vi "Reto2.vi"() -> ()   [LabVIEW 2018]
uses:
  <vilib>/Platform/TimedLoop/XDataNode/timing_clust.ctl
  <vilib>/Platform/TimedLoop/XDataNode/nitl_modes.ctl
  <vilib>/Platform/TimedLoop/XDataNode/wakeup.ctl
  <vilib>/platform/TimedLoop/XDataNode/XDataNode.xnode
  <vilib>/Platform/TimedLoop/XDataNode/XDNodeRunTimeDep.lvlib
panel:
  out "Waveform Chart":dbl(graph)
  in  "x":dbl min=0.0 max=100.0 step=10.0
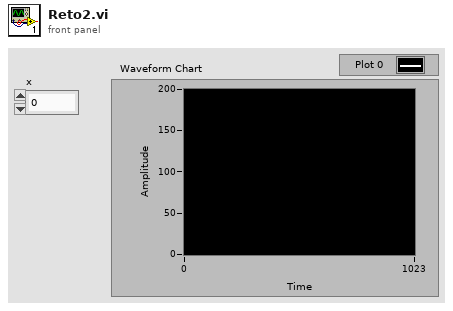
[diagram p1: front panel]
types:
  T1 = typedef "XDNodeRunTimeDep.lvlib/timing_clust.ctl" = cluster{"Expected End [f-1]":u64, "Actual End [f-1]":u64, "Finished Late? [f-1]":bool, "Expected End [i-1]":u64, "Actual End [i-1]":u64, "Finished Late? [i-1]":bool, "Expected Start [i]":u64, "Actual Start [i]":u64, "Expected Start [f]":u64, "Actual Start [f]":u64, "Source Name":string, "Structure Name":string, "Period":i64, "Deadline":i64, "Offset":i64, "Start":i64, "Priority":i32, "Timeout":i32, "Mode":T2, "Wakeup Reason":T3, "Error":errorcluster, "Source Type":string, "Secondary Source Type":string, "Global End Time":u64, "Global Start Time":u64, "Frame Duration":u64, "Iteration Duration":u64, "Assigned CPU":i32, "I/O Scan Engine Mode":u32}
  T2 = typedef "XDNodeRunTimeDep.lvlib/nitl_modes.ctl" = enum32{"No Change", "Process missed periods, maintain original phase", "Discard missed periods, maintain original phase", "Process missed periods, ignore original phase", "Discard missed periods, ignore original phase"}
  T3 = typedef "XDNodeRunTimeDep.lvlib/wakeup.ctl" = enum32{"Normal", "Aborted", "Asynchronous wakeup", "Timing source error", "Timed loop error", "Timeout"}
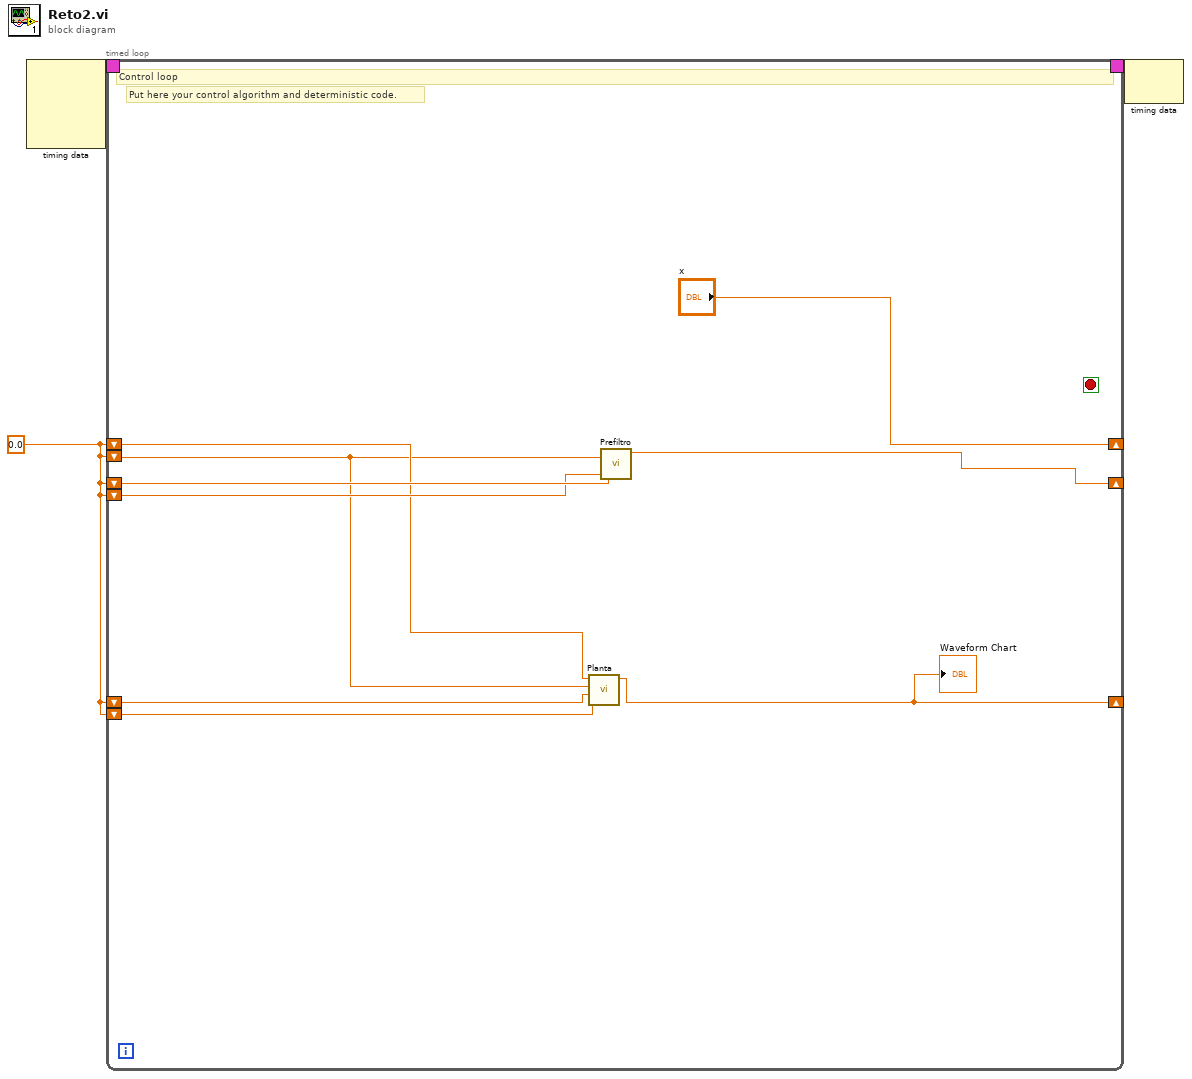
[diagram p0: block diagram]
diagram:
  w1 = 0.0 ("x")
  n1 = node-c288() -> (w3:T1)  [unwired: 4 in]
  n2 = timed-loop {
    timing: w3 -> [_]
    timing-out: [_] -> w2
    shift-right: ["x"] -> _
    shift-left: w1 -> [w8]
    shift-right: [w9] -> _
    shift-left: w1 -> [w11]
    shift-left: w1 -> [w7]
    shift-left: w1 -> [w10]
    shift-right: [w4] -> _
    shift-left: w1 -> [w6]
    shift-left: w1 -> [w5]
    stop <- _ stop-if-true
    # "Put here your control algorithm and deterministic code."
    # "Control loop"
    n3 = call "Planta.vi"("x_k-1"=w8, "x_k-2"=w7, "y_k-1"=w6, "y_k-2"=w5) -> ("y_k"=w4:dbl)  [unwired: 6 in]
    "Waveform Chart" <- w4
    n4 = call "Prefiltro.vi"("y_k-2"=w10, "y_k-1"=w11, "x_k-2"=w7) -> ("y_k"=w9:dbl)  [unwired: 5 in]
  }
  n5 = node-c288(w2) -> ()  [unwired: 1 out]
